vi "PH_ImageCoG_Plotter.PC Set Position Expectiation Values.vi"(0 "i ref in":refnum<vi>, 2 "expected X":i32, 3 "expected Y":i32, 5 "error in (no error)":errorcluster) -> (14 "i ref out":refnum<vi>, 19 "error out":errorcluster)   [LabVIEW 2014, in "PH_ImageCoG_Plotter.lvlib"]
doc: "This is the Action of the \"Set Position Expectiation values\"-Case: It sets the expectiation values for x- and y-position to own attributes and the GUI elements. This VI may be used elsewhere."
uses:
  PH_ImageCoG_Plotter.lvlib
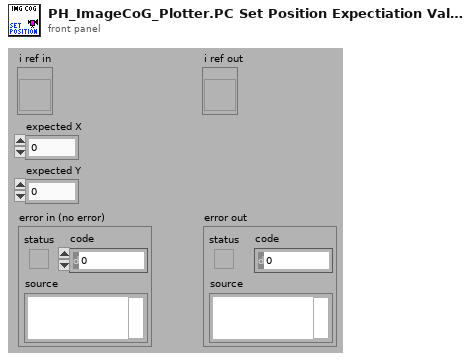
[diagram p1: front panel]
types:
  T1 = typedef "PH_ImageCoG_Plotter.lvlib/PH_ImageCoG_Plotter.i attribute.ctl" = cluster{"GUI Refs":cluster{"Delete":refnum<vi>, "Calibration status":refnum<vi>, "BI subtracted":refnum<vi>, "calc Beam Anal":refnum<vi>, "CoG - x":refnum<vi>, "CoG - y":refnum<vi>, "Type":refnum<vi>, "Center":refnum<vi>, "exp - X":refnum<vi>, "exp - Y":refnum<vi>, "Delta - X":refnum<vi>, "Delta - Y":refnum<vi>, "Available Cams":refnum<vi>, "CoG X":refnum<vi>, "CoG Y":refnum<vi>, "Delta X":refnum<vi>, "Delta Y":refnum<vi>, "Export Data":refnum<vi>, "Calibration data":refnum<vi>}, "Calibration":cluster{"Status":T2, "Calibration data":T3, "Calibration Data File":path}, "Beam Analysis":cluster{"on":bool, "exp - X":i32, "exp - Y":i32, "Type":bool, "Data":cluster{"current time":timestamp, "CoG-x":dbl, "CoG-y":dbl, "Delta-x":dbl, "Delta-y":dbl}[], "Datasets strored":i32, "Dataarray Size":i32}, "Cam instances":string[], "DIM Service Events":T4[], "Images":cluster{"Background":T7, "OP":T7, "GUI":T7}}
  T2 = typedef "PH_StatusHandler.lvlib/PH_StatusHandler.Status.ctl" = i16
  T3 = typedef "PH_ImageCalibrator.lvlib/PH_ImageCalibrator.Calibration Data.ctl" = cluster{"Date":string, "Time":string, "Cam Settings":cluster{"Cam ID":string, "Gain":dbl, "Brightness":dbl, "Shutter":dbl, "Cam Error":bool, "Mode":i32}, "Background Image":cluster{"Image":dbl[][], "Image Error":bool}, "Linear Calibration":cluster{"Calibration Factor":dbl, "not mm or mrad":bool}, "Energy Calibration":cluster{"Calibration Factor":dbl, "no mJ":bool}}
  T4 = typedef "BaseProcess.lvlib/BaseProcess.event definition.ctl" = cluster{"CAEEvtDef":T5, "Data Descriptor":T6}
  T5 = typedef "CAEObj.lvlib/CAEObj.event definition.ctl" = cluster{"URL":string, "enable":bool, "ignoreResID":bool}
  T6 = typedef "BaseProcess.lvlib/BaseProcess.descriptor string definition.ctl" = string
  T7 = typedef "IMAQ Image.ctl" = refnum<image>
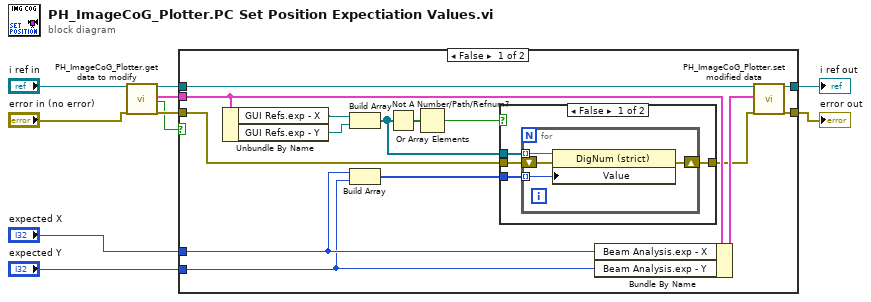
[diagram p0: block diagram]
diagram:
  n1 = call "PH_ImageCoG_Plotter.get data to modify.vi"("i ref in"="i ref in", "error in (no error)"="error in (no error)") -> ("i ref out"=w7:refnum<vi>, "i attribute"=w9:T1, "timed out"=w2:bool, "error out"=w5:errorcluster)  [unwired: 14 in]
  n2 = case shown="False" w2 {
    tunnel: "expected X" -> [w13 _]
    tunnel: w9 -> [w21 _]
    tunnel: [w24 w36] -> w8
    tunnel: w7 -> [w23 w36]
    tunnel: [w22 w35] -> w6
    tunnel: w5 -> [w20 w35]
    tunnel: "expected Y" -> [w12 _]
    frame False {
      n3 = Unbundle By Name(w21) -> ("GUI Refs.exp - X"=w18:refnum<vi>, "GUI Refs.exp - Y"=w15:refnum<vi>)
      n4 = Build Array(w18, w15) -> (w14:refnum<vi>[])
      n5 = Build Array(w13, w12) -> (w11:i32[])
      n6 = Not A Number/Path/Refnum?(number/path/refnum=w14) -> (NaN/Path/Refnum?=w17:bool[])
      n7 = Or Array Elements(Boolean array=w17) -> (logical OR=w16:bool)
      n8 = case shown="False" w16 {
        tunnel: w14 -> [w29 _]
        tunnel: w20 -> [w28 w34]
        tunnel: [w27 w34] -> w19
        tunnel: w11 -> [w26 _]
        frame False {
          n9 = for {
            tunnel: w29 -> [w33] mode=indexing
            shift-right: [w31] -> w27
            shift-left: w28 -> [w32]
            tunnel: w26 -> [w30] mode=indexing
            n10 = property class="DigNum (strict)"(reference=w33, error in=w32, "Value"=w30) -> (error out=w31:errorcluster)  [unwired: 1 out]
          }
        }
        frame True {
        }
      }
      n11 = Bundle By Name(cluster=w21, "Beam Analysis.exp - X"=w13, "Beam Analysis.exp - Y"=w12) -> (w25:T1)
      n12 = call "PH_ImageCoG_Plotter.set modified data.vi"("i ref in"=w23, "i attribute"=w25, "error in (no error)"=w19) -> ("i ref out"=w24:refnum<vi>, "error out"=w22:errorcluster)  [unwired: 15 in]
    }
    frame True {
    }
  }
  "i ref out" <- w8
  "error out" <- w6
